vi "LM Asymmetric Lorentzian and gradient.vi"(3 "output control":T1, 4 "data":variant, 5 "X":dbl[](array[numeric]), 6 "a":dbl[](array[numeric])) -> (0 "error out":errorcluster, 1 "f'(X,a)":dbl[][](array[numeric]), 2 "f(X,a)":dbl[](array[numeric]))   [LabVIEW 2021, in "Fits.lvlib"]
doc: "This template is the starting point for creating a model function to be passed to the Nonlinear Curve Fit.vi."
uses:
  <vilib>/gmath/NumericalOptimization/LM_output select.ctl
  Fits.lvlib
  <vilib>/gmath/NI_Gmath.lvlib
panel:
  # "Parameters:\n\namplitude: A\ncenter: t_0\nFWHM-: w-\nFWHM+: w+"
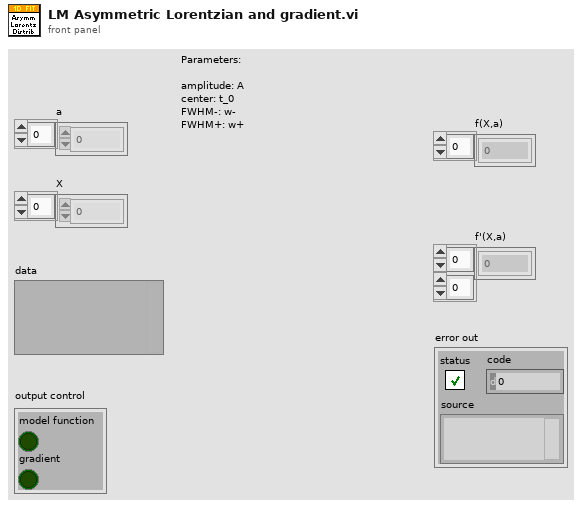
[diagram p1: front panel]
types:
  T1 = typedef "NI_Gmath.lvlib/LM_output select.ctl" = cluster{"model function":bool, "gradient":bool}
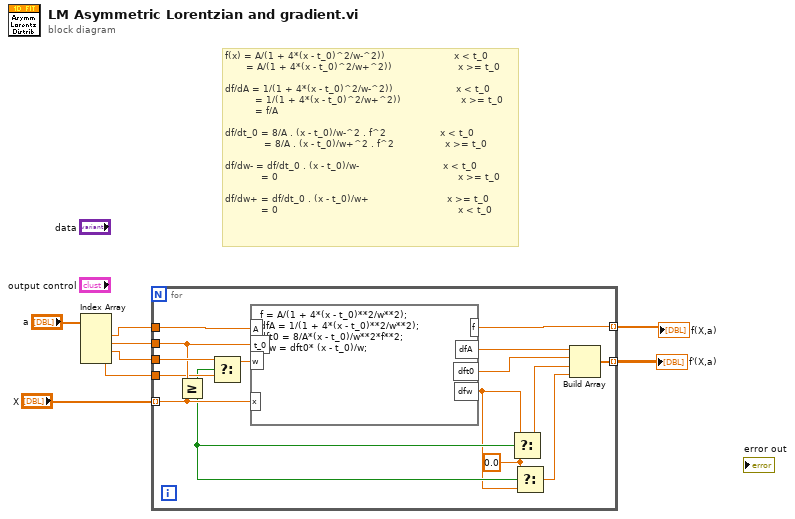
[diagram p0: block diagram]
diagram:
  # "f(x) = A/(1 + 4*(x - t_0)^2/w-^2))                       x < t_0\n       = A/(1 + 4*(x - t_0)^2/w+^2))                      x >= t_0\n\ndf/dA = 1/(1 + 4*(x - t_0)^2/w-^2))                     x < t_0\n          = 1/(1 + 4*(x - t_0)^2/w+^2))                    x >= t_0\n          = f/A\n\ndf/dt_0 = 8/A . (x - t_0)/w-^2 . f^2                  x < t_0\n             = 8/A . (x - t_0)/w+^2 . f^2                 x >= t_0\n\ndf/dw- = df/dt_0 . (x - t_0)/w-                            x < t_0\n            = 0                                                            x >= t_0\n\ndf/dw+ = df/dt_0 . (x - t_0)/w+                          x >= t_0\n            = 0                                                            x < t_0"
  n1 = Index Array(array="a") -> (element #1=w7:dbl, element #2=w6:dbl, element #3=w5:dbl, element #4=w4:dbl)  [unwired: 4 in]
  n2 = for {
    tunnel: w7 -> [w23]
    tunnel: w6 -> [w20]
    tunnel: w5 -> [w22]
    tunnel: w4 -> [w18]
    tunnel: "X" -> [w19] mode=indexing
    tunnel: [w13] -> w2 mode=indexing
    tunnel: [w9] -> w1 mode=indexing
    w16 = 0.0 ("f")
    n3 = Greater Or Equal?(x=w20, y=w19) -> (x >= y?=w17:bool)
    n4 = Select(t=w22, s=w17, f=w18) -> (s? t:f=w21:dbl)
    n5 = formula code="f = A/(1 + 4*(x - t_0)**2/w**2);\ndfA = 1/(1 + 4*(x - t_0)**2/w**2);\ndft0 = 8/A*(x - t_0)/w**2*f**2;\ndfw = dft0* (x - t_0)/w;"("A"=w23, "t_0"=w20, "w"=w21, "x"=w19) -> ("f"=w13:dbl, "dfA"=w14:dbl, "dft0"=w12:dbl, "dfw"=w15:dbl)
    n6 = Select(t=w15, s=w17, f=w16) -> (s? t:f=w11:dbl)
    n7 = Select(t=w16, s=w17, f=w15) -> (s? t:f=w10:dbl)
    n8 = Build Array(w14, w12, w11, w10) -> (w9:dbl[])
  }
  "f(X,a)" <- w2
  "f'(X,a)" <- w1
